vi "test-unscented-kalman-filter-ALL.vi"(8 "error in (no error)":errorcluster) -> (0 "error out":errorcluster, 3 "All Tests Passed":bool)   [LabVIEW 2019]
panel:
  out "Test 3":bool
  out "Test 2":bool
  out "Test 1":bool
  out "Test 0":bool
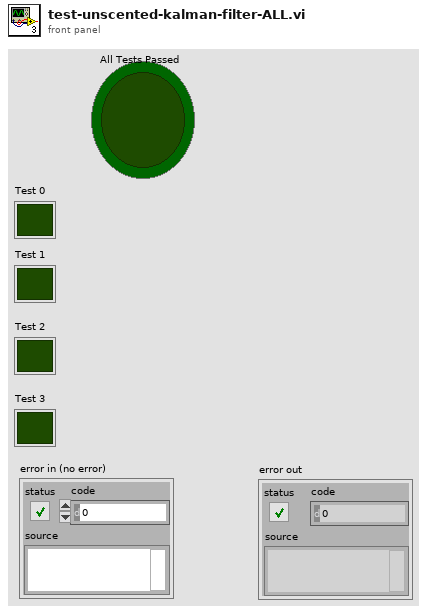
[diagram p1: front panel]
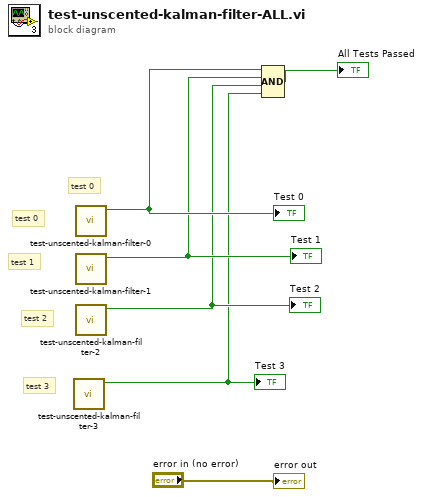
[diagram p0: block diagram]
diagram:
  # "test 3"
  # "test 0"
  # "test 2"
  # "test 1"
  # "test 0"
  n1 = call "test-unscented-kalman-filter-3.vi"() -> ("Test good"=w2:bool)  [unwired: 11 in]
  "Test 3" <- w2
  n2 = call "test-unscented-kalman-filter-0.vi"() -> ("All Tests Good"=w6:bool)  [unwired: 11 in]
  "Test 0" <- w6
  n3 = call "test-unscented-kalman-filter-1.vi"() -> ("Test good"=w5:bool)  [unwired: 11 in]
  "Test 1" <- w5
  n4 = call "test-unscented-kalman-filter-2.vi"() -> ("Test good"=w3:bool)  [unwired: 11 in]
  "Test 2" <- w3
  n5 = Compound Arithmetic op=AND(w6, w5, w3, w2) -> (→"All Tests Passed":bool)
  "error out" <- "error in (no error)"
